vi "Hadmard Matrix_Initialize.vi"(11 "matrix size":i32) -> (0 "error":i32, 2 "k [m*2^k=n]":i32, 3 "Initial Hadamard Matrix":i8[][](array[numeric]))   [LabVIEW 2014, in "NI_AALPro.lvlib"]
uses:
  NI_AALPro.lvlib
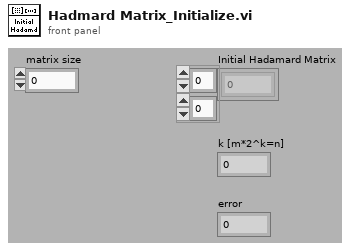
[diagram p1: front panel]
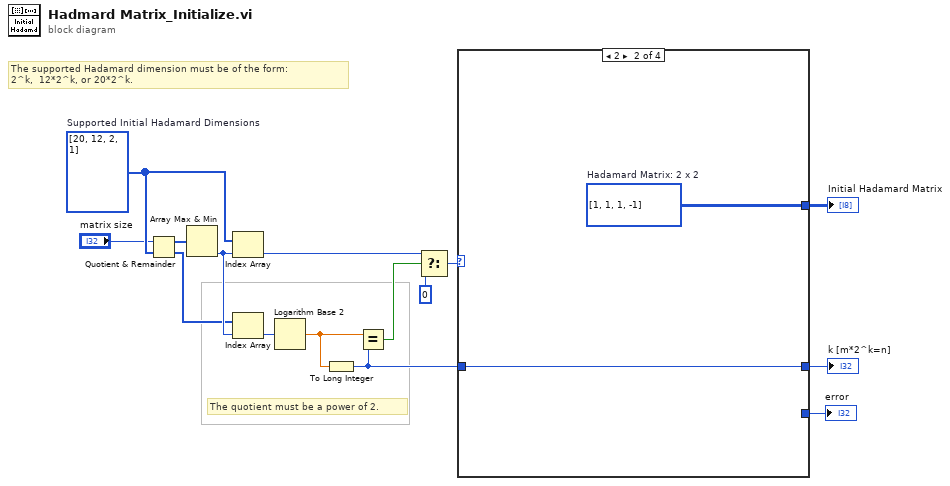
[diagram p0: block diagram]
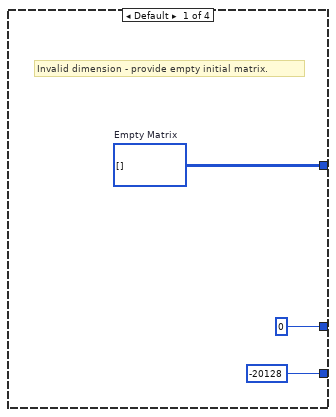
[diagram p2: hidden frame]
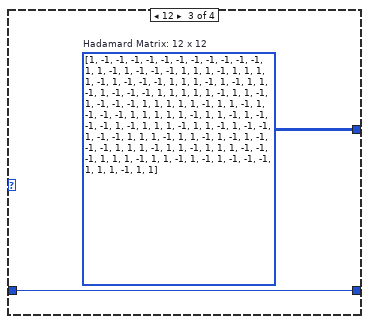
[diagram p3: hidden frame]
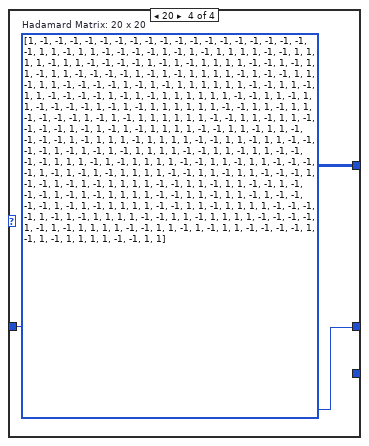
[diagram p4: hidden frame]
diagram:
  w15 = i32[] [20, 12, 2, 1]  # Supported Initial Hadamard Dimensions
  # "The supported Hadamard dimension must be of the form:\n2^k,  12*2^k, or 20*2^k."
  # "The quotient must be a power of 2."
  n1 = Quotient & Remainder(x="matrix size", y=w15) -> (x-y*floor(x/y)=w14:i32[], floor(x/y)=w8:i32[])
  n2 = Array Max & Min(array=w14) -> (min index (indices)=w12:i32)  [unwired: 3 out]
  n3 = Index Array(array=w15, index=w12) -> (element=w10:i32)
  n4 = Index Array(array=w8, index=w12) -> (element=w7:i32)
  n5 = Logarithm Base 2(1:w7) -> (0:w6:dbl)
  n6 = To Long Integer(number=w6) -> (32bit integer=w5:i32)
  n7 = Equal?(x=w6, y=w5) -> (x = y?=w2:bool)
  n8 = Select(t=w10, s=w2, f=0) -> (s? t:f=w11:i32)
  n9 = case shown="2" w11 {
    tunnel: [w18 w20 w22 w24] -> w13
    tunnel: w5 -> [_ w19 w21 w23]
    tunnel: [0 w19 w21 w23] -> w4
    tunnel: [-20128 _ _ _] -> w3
    frame Default {
      w18 = i8[][] []  # Empty Matrix
      # "Invalid dimension - provide empty initial matrix."
    }
    frame 2 {
      w20 = i8[][] [[1, 1], [1, -1]]  # Hadamard Matrix: 2 x 2
    }
    frame 12 {
      w22 = i8[][] [[1, -1, -1, -1, -1, -1, -1, -1, -1, -1, -1, -1], [1, 1, -1, 1, -1, -1, -1, 1, 1, 1, -1, 1], [1, 1, 1, -1, 1, -1, -1, -1, 1, 1, 1, -1], [1, -1, 1, 1, -1, 1, -1, -1, -1, 1, 1, 1], [1, 1, -1, 1, 1, -1, 1, -1, -1, -1, 1, 1], [1, 1, 1, -1, 1, 1, -1, 1, -1, -1, -1, 1], [1, 1, 1, 1, -1, 1, 1, -1, 1, -1, -1, -1], [1, -1, 1, 1, 1, -1, 1, 1, -1, 1, -1, -1], [1, -1, -1, 1, 1, 1, -1, 1, 1, -1, 1, -1], [1, -1, -1, -1, 1, 1, 1, -1, 1, 1, -1, 1], [1, 1, -1, -1, -1, 1, 1, 1, -1, 1, 1, -1], [1, -1, 1, -1, -1, -1, 1, 1, 1, -1, 1, 1]]  # Hadamard Matrix: 12 x 12
    }
    frame 20 {
      w24 = i8[][] [[1, -1, -1, -1, -1, -1, -1, -1, -1, -1, -1, -1, -1, -1, -1, -1, -1, -1, -1, -1], [1, 1, -1, 1, 1, -1, -1, -1, -1, 1, -1, 1, -1, 1, 1, 1, 1, -1, -1, 1], [1, 1, 1, -1, 1, 1, -1, -1, -1, -1, 1, -1, 1, -1, 1, 1, 1, 1, -1, -1], [1, -1, 1, 1, -1, 1, 1, -1, -1, -1, -1, 1, -1, 1, -1, 1, 1, 1, 1, -1], [1, -1, -1, 1, 1, -1, 1, 1, -1, -1, -1, -1, 1, -1, 1, -1, 1, 1, 1, 1], [1, 1, -1, -1, 1, 1, -1, 1, 1, -1, -1, -1, -1, 1, -1, 1, -1, 1, 1, 1], [1, 1, 1, -1, -1, 1, 1, -1, 1, 1, -1, -1, -1, -1, 1, -1, 1, -1, 1, 1], [1, 1, 1, 1, -1, -1, 1, 1, -1, 1, 1, -1, -1, -1, -1, 1, -1, 1, -1, 1], [1, 1, 1, 1, 1, -1, -1, 1, 1, -1, 1, 1, -1, -1, -1, -1, 1, -1, 1, -1], [1, -1, 1, 1, 1, 1, -1, -1, 1, 1, -1, 1, 1, -1, -1, -1, -1, 1, -1, 1], [1, 1, -1, 1, 1, 1, 1, -1, -1, 1, 1, -1, 1, 1, -1, -1, -1, -1, 1, -1], [1, -1, 1, -1, 1, 1, 1, 1, -1, -1, 1, 1, -1, 1, 1, -1, -1, -1, -1, 1], [1, 1, -1, 1, -1, 1, 1, 1, 1, -1, -1, 1, 1, -1, 1, 1, -1, -1, -1, -1], [1, -1, 1, -1, 1, -1, 1, 1, 1, 1, -1, -1, 1, 1, -1, 1, 1, -1, -1, -1], [1, -1, -1, 1, -1, 1, -1, 1, 1, 1, 1, -1, -1, 1, 1, -1, 1, 1, -1, -1], [1, -1, -1, -1, 1, -1, 1, -1, 1, 1, 1, 1, -1, -1, 1, 1, -1, 1, 1, -1], [1, -1, -1, -1, -1, 1, -1, 1, -1, 1, 1, 1, 1, -1, -1, 1, 1, -1, 1, 1], [1, 1, -1, -1, -1, -1, 1, -1, 1, -1, 1, 1, 1, 1, -1, -1, 1, 1, -1, 1], [1, 1, 1, -1, -1, -1, -1, 1, -1, 1, -1, 1, 1, 1, 1, -1, -1, 1, 1, -1], [1, -1, 1, 1, -1, -1, -1, -1, 1, -1, 1, -1, 1, 1, 1, 1, -1, -1, 1, 1]]  # Hadamard Matrix: 20 x 20
    }
  }
  "Initial Hadamard Matrix" <- w13
  "k [m*2^k=n]" <- w4
  "error" <- w3
